vi "peak comb -- interpolate V0.vi"(6 "all peaks exp":i32[](array[numeric])=[564, 649, 987, 1133, 1214, 1585, 1763, 1823, 1880, 1899, 2032, 2138, 2221, 2270, 2350, 2456, 2580, 2634, 2831, 2960, 2965, 3131, 3328, 3469, 3553, 0, 3615, 3734, 0, 0, 0, 4236, 4300, 4331], 8 "Gamma":dbl, 11 "freq":dbl) -> (3 "Numeric":dbl)   [LabVIEW 2010]
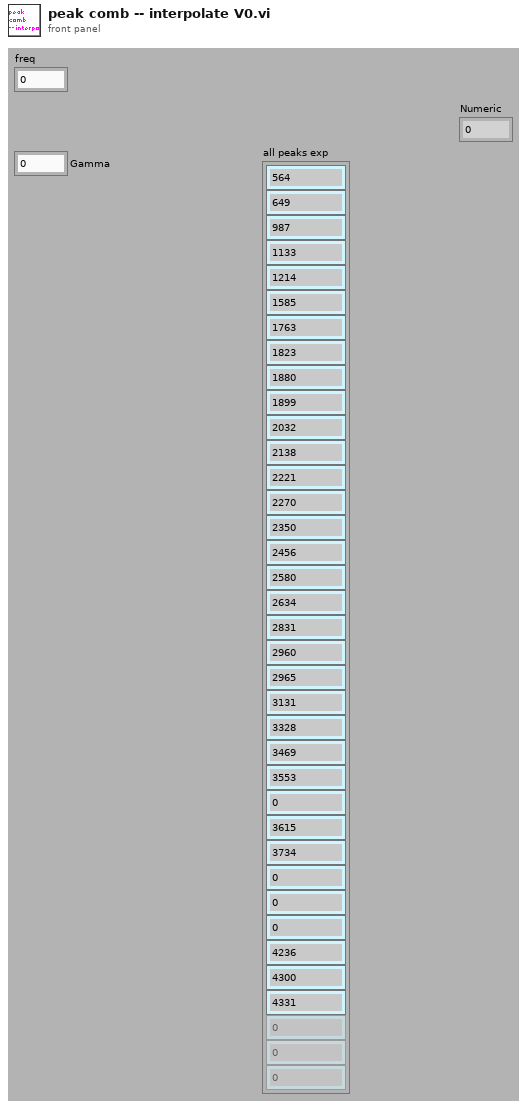
[diagram p1: front panel]
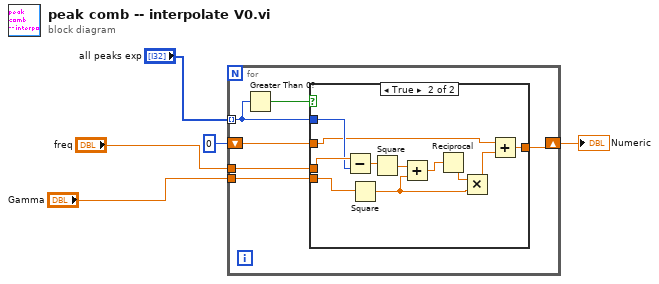
[diagram p0: block diagram]
diagram:
  n1 = for {
    tunnel: "all peaks exp" -> [w7] mode=indexing
    tunnel: "freq" -> [w11]
    tunnel: "Gamma" -> [w10]
    shift-right: [w8] -> w1
    shift-left: 0 -> [w9]
    n2 = Greater Than 0?(x=w7) -> (x > 0?=w6:bool)
    n3 = case shown="True" w6 {
      tunnel: w11 -> [_ w23]
      tunnel: w7 -> [_ w22]
      tunnel: w10 -> [_ w19]
      tunnel: w9 -> [w12 w18]
      tunnel: [w12 w17] -> w8
      frame False {
      }
      frame True {
        n4 = Subtract(x=w23, y=w22) -> (x-y=w21:dbl)
        n5 = Square(x=w19) -> (x^2=w14:dbl)
        n6 = Square(x=w21) -> (x^2=w20:dbl)
        n7 = Add(x=w20, y=w14) -> (x+y=w16:dbl)
        n8 = Reciprocal(x=w16) -> (1/x=w15:dbl)
        n9 = Multiply(x=w15, y=w14) -> (x*y=w13:dbl)
        n10 = Add(x=w18, y=w13) -> (x+y=w17:dbl)
      }
    }
  }
  "Numeric" <- w1
